vi "Configure Bus Source (CAN).vi"(0 "VISA resource name":refnum<visa-resource-name>, 1 "Bit Rate (2: 500 Kbps)":u16(ring)=2 items=["1 Mbps", "800 Kbps", "500 Kbps", "250 Kbps", "125 Kbps", "100 Kbps", "92.2 Kbps", "83.3 Kbps", "62.5 Kbps", "50 Kbps", "37 Kbps", "33.3 Kbps", "20 Kbps", "10 Kbps", "Custom"], 5 "BUS Number (9: Bus 1)":u16(ring)=9 items=["Bus 1"=9, "Bus 2"=10, "Bus 3"=11, "Bus 4"=12], 7 "Source (0: Channel 1)":u16(ring) items=["Channel 1"=0, "Channel 2"=1, "Channel 3"=2, "Channel 4"=3, "Digital Channel 0"=14, "Digital Channel 1"=15, "Digital Channel 2"=16, "Digital Channel 3"=17, "Digital Channel 4"=18, "Digital Channel 5"=19, "Digital Channel 6"=20, "Digital Channel 7"=21, "Digital Channel 8"=22, "Digital Channel 9"=23, "Digital Channel 10"=24, "Digital Channel 11"=25, "Digital Channel 12"=26, "Digital Channel 13"=27, "Digital Channel 14"=28, "Digital Channel 15"=29], 9 "Signal Type (0: CAN High)":u16(ring) items=["CAN High", "CAN Low", "Rx", "Tx", "Differential"], 11 "error in (no error)":errorcluster, 12 "Custom Bitrate (500000 bps)":dbl=500000.0, 13 "Sampling Point (50 %)":dbl=50.0) -> (4 "VISA resource name out":refnum<visa-resource-name>, 15 "error out":errorcluster)   [LabVIEW 2009, in "Tektronix DPO MSO 2000 4000 Series.lvlib"]
doc: "Configures CAN bus settings for an oscilloscope."
uses:
  <instrlib>/Tektronix DPO MSO 2000 4000 Series/Tektronix DPO MSO 2000 4000 Series.lvlib
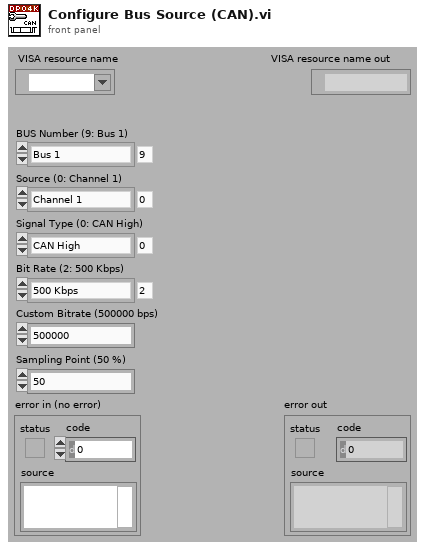
[diagram p1: front panel]
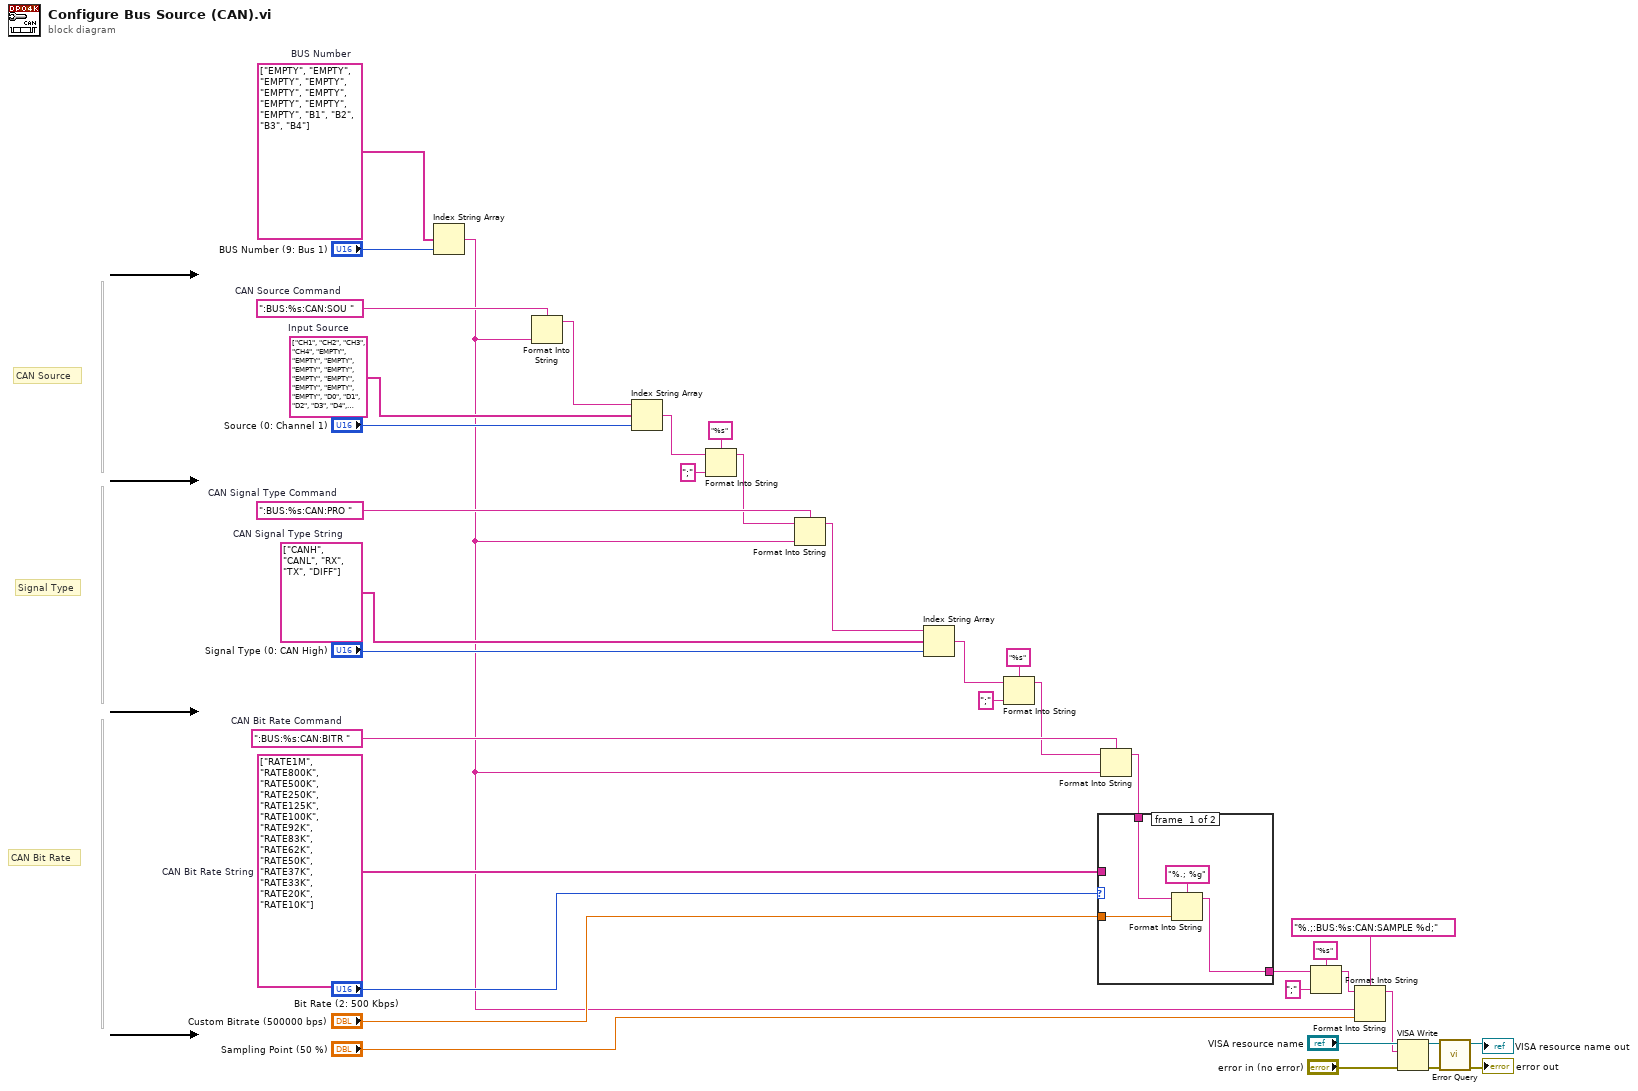
[diagram p0: block diagram]
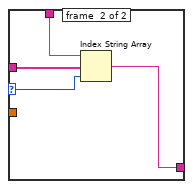
[diagram p2: hidden frame]
diagram:
  w12 = string[] ["RATE1M", "RATE800K", "RATE500K", "RATE250K", "RATE125K", "RATE100K", "RATE92K", "RATE83K", "RATE62K", "RATE50K", "RATE37K", "RATE33K", "RATE20K", "RATE10K"]  # CAN Bit Rate String
  w26 = string[] ["CANH", "CANL", "RX", "TX", "DIFF"]  # CAN Signal Type String
  w31 = ":BUS:%s:CAN:PRO "  # CAN Signal Type Command
  w25 = ":BUS:%s:CAN:BITR "  # CAN Bit Rate Command
  w34 = ":BUS:%s:CAN:SOU "  # CAN Source Command
  w27 = string[] ["CH1", "CH2", "CH3", "CH4", "EMPTY", "EMPTY", "EMPTY", "EMPTY", "EMPTY", "EMPTY", "EMPTY", "EMPTY", "EMPTY", "EMPTY", "D0", "D1", "D2", "D3", "D4", "D5", "D6", "D7", "D8", "D9", "D10", "D11", "D12", "D13", "D14", "D15"]  # Input Source
  w36 = string[] ["EMPTY", "EMPTY", "EMPTY", "EMPTY", "EMPTY", "EMPTY", "EMPTY", "EMPTY", "EMPTY", "B1", "B2", "B3", "B4"]  # BUS Number
  # "CAN Bit Rate"
  # "Signal Type"
  # "CAN Source"
  n1 = Index String Array(1:"BUS Number (9: Bus 1)", 2:w36) -> (0:w1:string)  [unwired: 1 in]
  n2 = Format Into String(format string=w34, w1) -> (resulting string=w33:string)  [unwired: 2 in, 1 out]
  n3 = Index String Array(1:"Source (0: Channel 1)", 2:w27, 3:w33) -> (0:w18:string)
  n4 = Format Into String(format string="%s", initial string=w18, ";" ("input 1")) -> (resulting string=w30:string)  [unwired: 1 in, 1 out]
  n5 = Format Into String(format string=w31, initial string=w30, w1) -> (resulting string=w28:string)  [unwired: 1 in, 1 out]
  n6 = Index String Array(1:"Signal Type (0: CAN High)", 2:w26, 3:w28) -> (0:w16:string)
  n7 = Format Into String(format string="%s", initial string=w16, ";" ("input 1")) -> (resulting string=w23:string)  [unwired: 1 in, 1 out]
  n8 = Format Into String(format string=w25, initial string=w23, w1) -> (resulting string=w22:string)  [unwired: 1 in, 1 out]
  n9 = case shown="0..13" "Bit Rate (2: 500 Kbps)" {
    selector: "Bit Rate (2: 500 Kbps)" -> [_ w42]
    tunnel: w22 -> [w41 w45]
    tunnel: [w38 w44] -> w14
    tunnel: w12 -> [_ w43]
    tunnel: "Custom Bitrate (500000 bps)" -> [w40 _]
    frame #0 {
      n10 = Format Into String(format string="%.; %g", initial string=w41, w40) -> (resulting string=w38:string)  [unwired: 1 in, 1 out]
    }
    frame #1 {
      n11 = Index String Array(1:w42, 2:w43, 3:w45) -> (0:w44:string)
    }
  }
  n12 = Format Into String(format string="%s", initial string=w14, ";" ("input 1")) -> (resulting string=w5:string)  [unwired: 1 in, 1 out]
  n13 = Format Into String(format string="%.;:BUS:%s:CAN:SAMPLE %d;", initial string=w5, w1, "Sampling Point (50 %)") -> (resulting string=w4:string)  [unwired: 1 in, 1 out]
  n14 = VISA Write(VISA resource name="VISA resource name", write buffer=w4, error in (no error)="error in (no error)") -> (VISA resource name out=w20:refnum<visa-resource-name>, error out=w19:errorcluster)  [unwired: 1 out]
  n15 = call <instrlib>:"Error Query.vi"("error in (no error)"=w19, "VISA resource name"=w20) -> ("error out"=→"error out":errorcluster, "VISA resource name out"=→"VISA resource name out":refnum<visa-resource-name>)  [unwired: 6 in, 2 out]
